vi "Boiler Controller.vi"(8 "error in":errorcluster, 10 "Notifiers":T1, 11 "Message Queues":T2) -> (0 "error out":errorcluster)   [LabVIEW 2015]
uses:
  support/Message Queue/All Message Queues.ctl
  support/Message Queue/Message Cluster.ctl
  support/Notifiers/Notifier.ctl
  support/Message Queue/Message Queue.lvlib
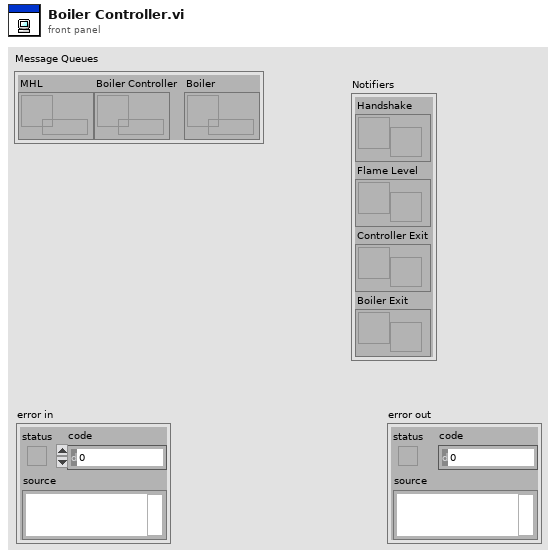
[diagram p1: front panel]
types:
  T1 = typedef "Notifier.ctl" = cluster{"Handshake":refnum<notifier>, "Flame Level":refnum<notifier>, "Controller Exit":refnum<notifier>, "Boiler Exit":refnum<notifier>}
  T2 = typedef "Message Queue.lvlib/All Message Queues.ctl" = cluster{"MHL":refnum<queue>, "Boiler Controller":refnum<queue>, "Boiler ":refnum<queue>}
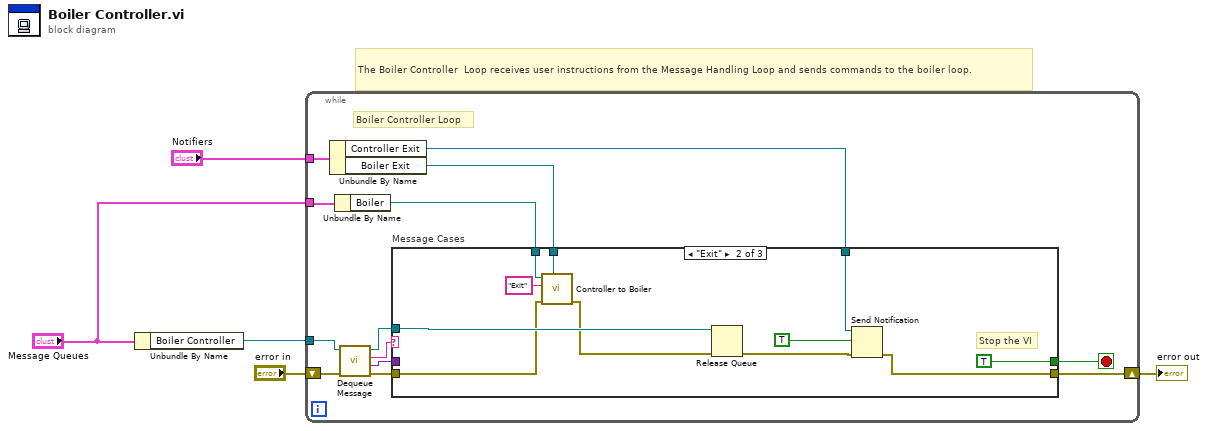
[diagram p0: block diagram]
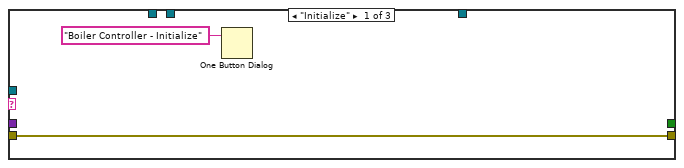
[diagram p2: hidden frame]
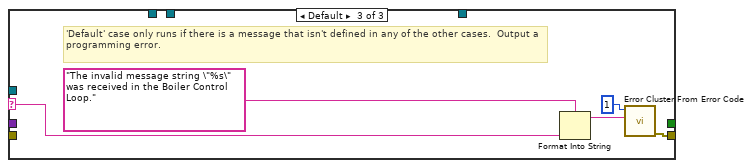
[diagram p3: hidden frame]
diagram:
  # "The Boiler Controller  Loop receives user instructions from the Message Handling Loop and sends commands to the boiler loop."
  n1 = Unbundle By Name("Message Queues") -> ("Boiler Controller"=w3:refnum<queue>)
  n2 = while {
    tunnel: w3 -> [w12]
    shift-right: [w11] -> w5
    shift-left: "error in" -> [w17]
    tunnel: "Notifiers" -> [w10]
    tunnel: "Message Queues" -> [w9]
    stop <- w18 stop-if-true
    # "Boiler Controller Loop"
    n3 = Unbundle By Name(w10) -> ("Controller Exit"=w6:refnum<notifier>, "Boiler Exit"=w7:refnum<notifier>)
    n4 = Unbundle By Name(w9) -> ("Boiler"=w8:refnum<queue>)
    n5 = call "Dequeue Message.vi"("error in (no error)"=w17, "Message Queue"=w12) -> ("error out"=w16:errorcluster, "Message Data"=w14:variant, "Message"=w15:string, "dup Message Queue"=w13:refnum<queue>)  [unwired: 6 in]
    n6 = case "Message Cases" shown="\"Exit\"" w15 {
      selector: w15 -> [_ _ w33]
      tunnel: w13 -> [_ w30 _]
      tunnel: w16 -> [w20 w26 _]
      tunnel: [w20 w24 w32] -> w11
      tunnel: [_ TRUE _] -> w18
      tunnel: w14 -> [_ _ _]
      tunnel: w8 -> [_ w28 _]
      tunnel: w7 -> [_ w27 _]
      tunnel: w6 -> [_ w21 _]
      frame "Initialize" {
        n7 = One Button Dialog(message="Boiler Controller - Initialize") -> ()  [unwired: 1 in, 1 out]
      }
      frame "Exit" {
        # "Stop the VI"
        n8 = call "Controller to Boiler.vi"("Notifier"=w27, "error in"=w26, "Message"="Exit", "Boiler Queue in"=w28) -> ("error out"=w25:errorcluster)  [unwired: 5 in, 2 out]
        n9 = Release Queue(queue=w30, error in (no error)=w25) -> (error out=w23:errorcluster)  [unwired: 1 in, 2 out]
        n10 = Send Notification(notification=TRUE, notifier=w21, error in (no error)=w23) -> (error out=w24:errorcluster)  [unwired: 1 out]
      }
      frame Default {
        # "'Default' case only runs if there is a message that isn't defined in any of the other cases.  Output a programming error."
        n11 = Format Into String(format string="The invalid message string \"%s\" was received in the Boiler Control Loop." ("Unknown Message Error Text"), w33) -> (resulting string=w34:string)  [unwired: 2 in, 1 out]
        n12 = call <vilib>:"Error Cluster From Error Code.vi"("error message (\"\")"=w34, "error code (0)"=1) -> ("error out"=w32:errorcluster)  [unwired: 7 in]
      }
    }
  }
  "error out" <- w5
